vi "Networking String Usecase.vi"() -> ()   [LabVIEW 2015]
panel:
  in  "data in":string
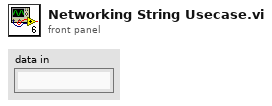
[diagram p1: front panel]
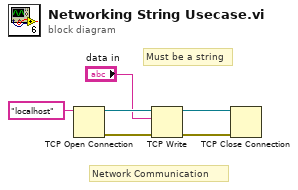
[diagram p0: block diagram]
diagram:
  # "Must be a string"
  # "Network Communication"
  n1 = TCP Open Connection(address="localhost") -> (connection ID=w6:refnum<k5>, error out=w5:errorcluster)  [unwired: 4 in]
  n2 = TCP Write(connection ID=w6, data in="data in", error in (no error)=w5) -> (connection ID out=w4:refnum<k5>, error out=w3:errorcluster)  [unwired: 1 in, 1 out]
  n3 = TCP Close Connection(connection ID=w4, error in (no error)=w3) -> ()  [unwired: 1 in, 2 out]
